vi "Configure CCDF.vi"(7 "X-axis Max Value (50 dB)":dbl=50.0, 8 "error in (no error)":errorcluster, 9 "Cumulative Count (8E+7)":dbl=80000000.0, 10 "CCDF Continuous Refresh (T: Enable)":bool=TRUE, 11 "VISA resource name":refnum<visa-resource-name>) -> (0 "error out":errorcluster, 3 "VISA resource name out":refnum<visa-resource-name>)   [LabVIEW 2018, in "Agilent U2000 Series.lvlib"]
doc: "Configures the settings of the Complementary Cumulative Distribution Function (CCDF), both in table and trace format.\n\nNote: \nThis VI is not applicable for U2040 X-Series."
uses:
  Agilent U2000 Series.lvlib
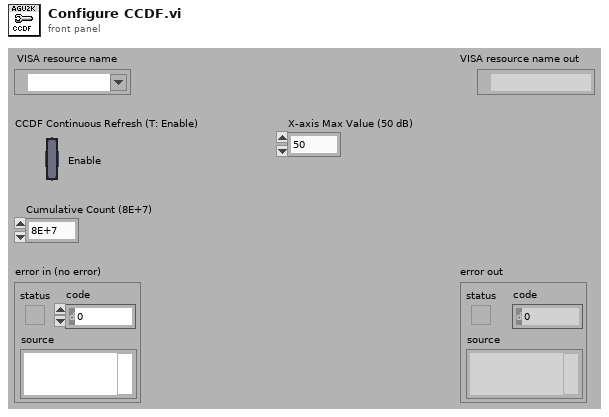
[diagram p1: front panel]
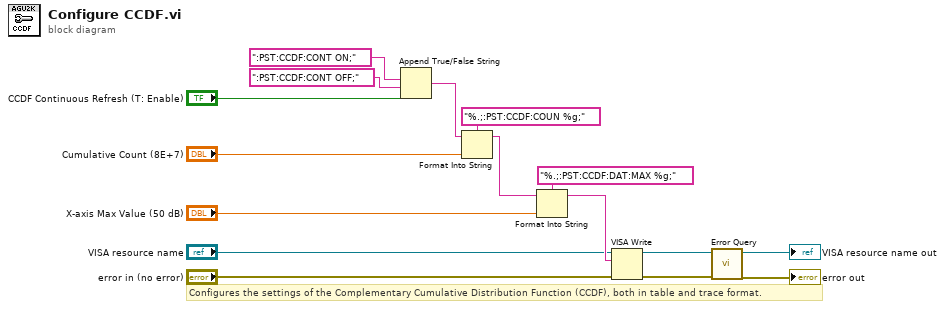
[diagram p0: block diagram]
diagram:
  # "Configures the settings of the Complementary Cumulative Distribution Function (CCDF), both in table and trace format."
  n1 = Append True/False String(1:"CCDF Continuous Refresh (T: Enable)", 2:":PST:CCDF:CONT OFF;", 3:":PST:CCDF:CONT ON;") -> (0:w13:string)  [unwired: 1 out]
  n2 = Format Into String(format string="%.;:PST:CCDF:COUN %g;", initial string=w13, "Cumulative Count (8E+7)") -> (resulting string=w10:string)  [unwired: 1 in, 1 out]
  n3 = Format Into String(format string="%.;:PST:CCDF:DAT:MAX %g;", initial string=w10, "X-axis Max Value (50 dB)") -> (resulting string=w7:string)  [unwired: 1 in, 1 out]
  n4 = VISA Write(VISA resource name="VISA resource name", write buffer=w7, error in (no error)="error in (no error)") -> (VISA resource name out=w4:refnum<visa-resource-name>, error out=w3:errorcluster)  [unwired: 1 out]
  n5 = call "Error Query.vi"("error in (no error)"=w3, "VISA resource name"=w4) -> ("error out"=→"error out":errorcluster, "VISA resource name out"=→"VISA resource name out":refnum<visa-resource-name>)  [unwired: 8 out]
